vi "Run Bfr Rx - Cached - Copy Cache.vi"(5 "Cache Buffer":u64 format="%016x", 7 "External Buffer":u64 format="%016x", 8 "error in (no error)":errorcluster, 11 "Temp Data in":u8[](array[numeric])) -> (0 "error out":errorcluster)   [LabVIEW 2019, in "UDP-Custom-Device Engine.lvlib"]
uses:
  UDP-Custom-Device Engine.lvlib
  <vilib>/NI VeriStand/VeriStand Data/Pointer Operations/Pointer.In-Place Read (1D U8).vi
  <vilib>/NI VeriStand/VeriStand Data/Pointer Operations/Pointer.Write (1D U8).vi
  <vilib>/NI VeriStand/VeriStand Data/VeriStand Data.lvlib
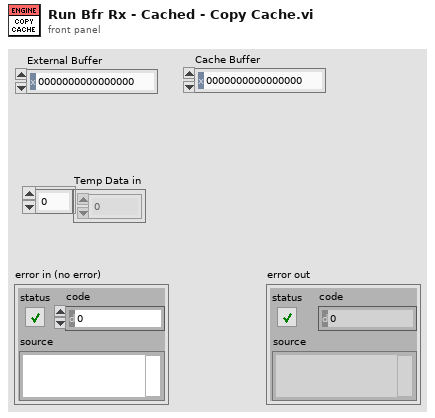
[diagram p1: front panel]
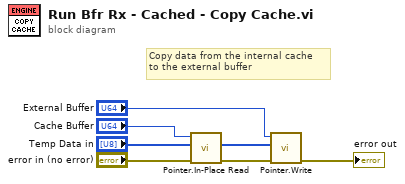
[diagram p0: block diagram]
diagram:
  # "Copy data from the internal cache\nto the external buffer"
  n1 = call-poly <vilib>:"Pointer.In-Place Read.vi"("error in (no error)"="error in (no error)", "allocated array in"="Temp Data in", "pointer in"="Cache Buffer") -> ("error out"=w6:errorcluster, "array out"=w3:u8[])  [unwired: 6 in, 1 out]
  n2 = call-poly <vilib>:"Pointer.Write.vi"("error in (no error)"=w6, "values"=w3, "pointer in"="External Buffer") -> ("error out"=→"error out":errorcluster)  [unwired: 6 in, 2 out]
